vi "E14_Global_Variable_1.1.vi"() -> ()   [LabVIEW 2020]
uses:
  Global 1.vi
panel:
  out "Numero a pasar":i32
  in  "Boton1":bool
  out "LED1":bool=TRUE
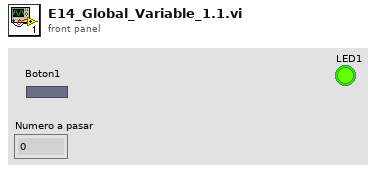
[diagram p1: front panel]
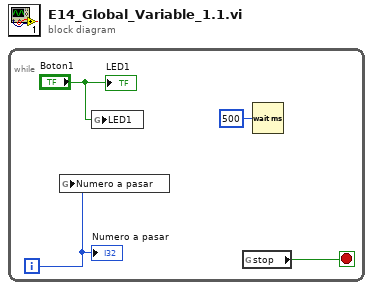
[diagram p0: block diagram]
diagram:
  n1 = while {
    i -> [w3]
    stop <- w1 stop-if-true
    n2 = global write "Global 1.vi" "Numero a pasar"(w3) -> ()
    n3 = global write "Global 1.vi" "LED1"("Boton1") -> ()
    n4 = global read "Global 1.vi" "stop"() -> (w1:bool)
    n5 = Wait (ms)(milliseconds to wait=u32 500) -> ()  [unwired: 1 out]
    "LED1" <- "Boton1"
    "Numero a pasar" <- w3
  }
